vi "porta_w_r.vi"() -> ()   [LabVIEW 2020]
uses:
  <vilib>/Instr/_visa.llb/VISA Configure Serial Port (Instr).vi
panel:
  out "read buffer":string
  in  "Numeric":dbl
  in  "VISA resource name":refnum<visa-resource-name>
  in  "String":string
  in  "stop":bool
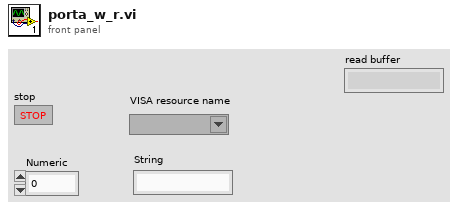
[diagram p1: front panel]
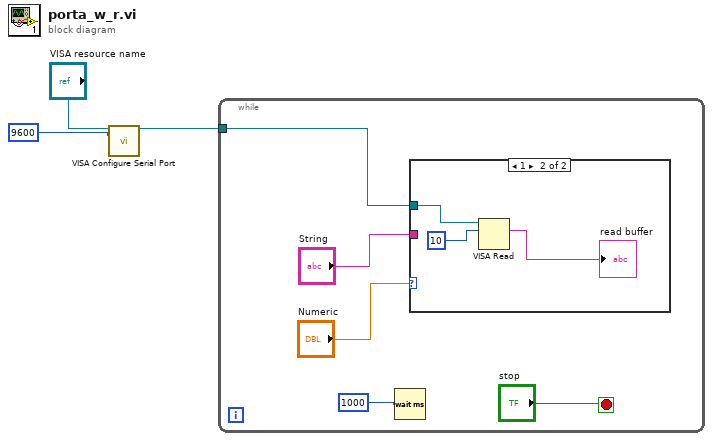
[diagram p0: block diagram]
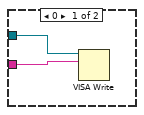
[diagram p2: hidden frame]
diagram:
  n1 = call-poly "VISA Configure Serial Port"("VISA resource name"="VISA resource name", "baud rate (9600)"=u32 9600) -> ("VISA resource name out"=w2:refnum<visa-resource-name>)  [unwired: 12 in, 1 out]
  n2 = while {
    tunnel: w2 -> [w6]
    stop <- "stop" stop-if-true
    n3 = Wait (ms)(milliseconds to wait=u32 1000) -> ()  [unwired: 1 out]
    n4 = case shown="1" "Numeric" {
      tunnel: "String" -> [w10 _]
      tunnel: w6 -> [w9 w13]
      frame 0 {
        n5 = VISA Write(VISA resource name=w9, write buffer=w10) -> ()  [unwired: 1 in, 3 out]
      }
      frame 1 {
        n6 = VISA Read(VISA resource name=w13, byte count=u32 10) -> (read buffer=→"read buffer":string)  [unwired: 1 in, 3 out]
      }
    }
  }
